vi "Read-Write Program File.vi"(0 "configuration file path":path=path "C:/ProgramData/PVI Systems/Vision Inspection System/Config.ini", 1 "Program in":T2={"Raw Logging Configuration"={"Log File Base Path"=path "", "Enable Log File"=FALSE}, "Sequence"={"Start RPM"=10.0, "End RPM"=9600.0, "# RPM Steps"=1, "Dwell (s)"=2.0, "Start L-value / Resist"=0, "End L-value/Resist"=0, "# L-value/Resist Steps"=0, "Steady State +/-RPM"=10.0, "Enable Steady State +/- RPM"=FALSE, "Steady State Window (s)"=10.0, "Enable Steady State Max Wait"=FALSE, "Max Settle Time (s)"=10.0, "Enable Temperature Rest"=FALSE, "Rest TC2 threshold (degF)"=2.0, "Enable Max Time Rest"=FALSE, "Max Rest Time (s)"=10.0, "Rest RPM"=2.0, "RPM Ramp (rpm/s)"=10.0, "Resistance Motor Mode"=enum."v1 Bike"}, "Summary  CSV Log Configuration"={"Report  CSV File Path"=path "C:/Users/nlim/Documents/LabVIEW Data/Logged Data.tdms", "Enable Report CSV File"=FALSE}, "CSV Log Info"={"Report Title"="", "Time Stamp"=timestamp(0 s since 1904-01-01), "Serial Number"="", "Initial Temperature"=0.0, "Comments"=""}, "Table"=[]} {"Sequence"."RPM Ramp (rpm/s)" min=0.0 format="%#_6f"; "Sequence"."Rest RPM" min=0.0 format="%.1f"; "Sequence"."Max Rest Time (s)" min=0.0 format="%.1f"; "Sequence"."Rest TC2 threshold (degF)" format="%.1f"; "Sequence"."Max Settle Time (s)" min=0.0 format="%.1f"; "Sequence"."Steady State Window (s)" min=0.0 format="%.1f"; "Sequence"."Steady State +/-RPM" min=0.0 format="%.1f"; "Sequence"."# L-value/Resist Steps" min=1; "Sequence"."End L-value/Resist" min=0 max=100; "Sequence"."Start L-value / Resist" min=0 max=100; "Sequence"."Dwell (s)" min=0.0 format="%#_6f"; "Sequence"."# RPM Steps" min=1; "Sequence"."End RPM" min=0.0 max=200.0 format="%#_6f"; "Sequence"."Start RPM" min=0.0 max=200.0 format="%#_6f"}, 2 "Mode":T1=enum."Write", 3 "error in":errorcluster) -> (7 "Config File Path":path=path "C:/ProgramData/PVI Systems/Vision Inspection System/Config.ini", 8 "Program out":T2={"Raw Logging Configuration"={"Log File Base Path"=path "", "Enable Log File"=FALSE}, "Sequence"={"Start RPM"=10.0, "End RPM"=9600.0, "# RPM Steps"=1, "Dwell (s)"=2.0, "Start L-value / Resist"=0, "End L-value/Resist"=0, "# L-value/Resist Steps"=0, "Steady State +/-RPM"=10.0, "Enable Steady State +/- RPM"=FALSE, "Steady State Window (s)"=10.0, "Enable Steady State Max Wait"=FALSE, "Max Settle Time (s)"=10.0, "Enable Temperature Rest"=FALSE, "Rest TC2 threshold (degF)"=2.0, "Enable Max Time Rest"=FALSE, "Max Rest Time (s)"=10.0, "Rest RPM"=2.0, "RPM Ramp (rpm/s)"=10.0, "Resistance Motor Mode"=enum."v1 Bike"}, "Summary  CSV Log Configuration"={"Report  CSV File Path"=path "C:/Users/nlim/Documents/LabVIEW Data/Logged Data.tdms", "Enable Report CSV File"=FALSE}, "CSV Log Info"={"Report Title"="", "Time Stamp"=timestamp(0 s since 1904-01-01), "Serial Number"="", "Initial Temperature"=0.0, "Comments"=""}, "Table"=[]} {"Sequence"."RPM Ramp (rpm/s)" min=0.0 format="%#_6f"; "Sequence"."Rest RPM" min=0.0 format="%.1f"; "Sequence"."Max Rest Time (s)" min=0.0 format="%.1f"; "Sequence"."Rest TC2 threshold (degF)" format="%.1f"; "Sequence"."Max Settle Time (s)" min=0.0 format="%.1f"; "Sequence"."Steady State Window (s)" min=0.0 format="%.1f"; "Sequence"."Steady State +/-RPM" min=0.0 format="%.1f"; "Sequence"."# L-value/Resist Steps" min=1; "Sequence"."End L-value/Resist" min=0 max=100; "Sequence"."Start L-value / Resist" min=0 max=100; "Sequence"."Dwell (s)" min=0.0 format="%#_6f"; "Sequence"."# RPM Steps" min=1; "Sequence"."End RPM" min=0.0 max=200.0 format="%#_6f"; "Sequence"."Start RPM" min=0.0 max=200.0 format="%#_6f"}, 10 "error out":errorcluster)   [LabVIEW 2015, in "Config Module.lvlib"]
uses:
  Config Module.lvlib
  Settings/Program Cluster.ctl
  Logging/Logging Configuration.ctl
  Settings/Sequence Cluster.ctl
  Resistance Motor/Resistance Mode Enum.ctl
  controls/CSV Log Cluster.ctl
  controls/CSV Log Info Cluster.ctl
  Controls/Config File Operation Enum.ctl
  XML Config/XML Config.lvlib
  Logging/Logging.lvlib
  Settings/Settings.lvlib
panel:
  # "Settled when"
  # "RPM is within"
  # "RPM of set RPM for last"
  # "seconds"
  # "OR"
  # "seconds since last step change"
  # "More than"
  # "Rest at end of each step at"
  # "RPM until"
  # "TC2 temperature is below"
  # "deg F"
  # "OR"
  # "seconds have elapsed"
  # "More than"
  # "Settled when"
  # "RPM is within"
  # "RPM of set RPM for last"
  # "seconds"
  # "OR"
  # "seconds since last step change"
  # "More than"
  # "Rest at end of each step at"
  # "RPM until"
  # "TC2 temperature is below"
  # "deg F"
  # "OR"
  # "seconds have elapsed"
  # "More than"
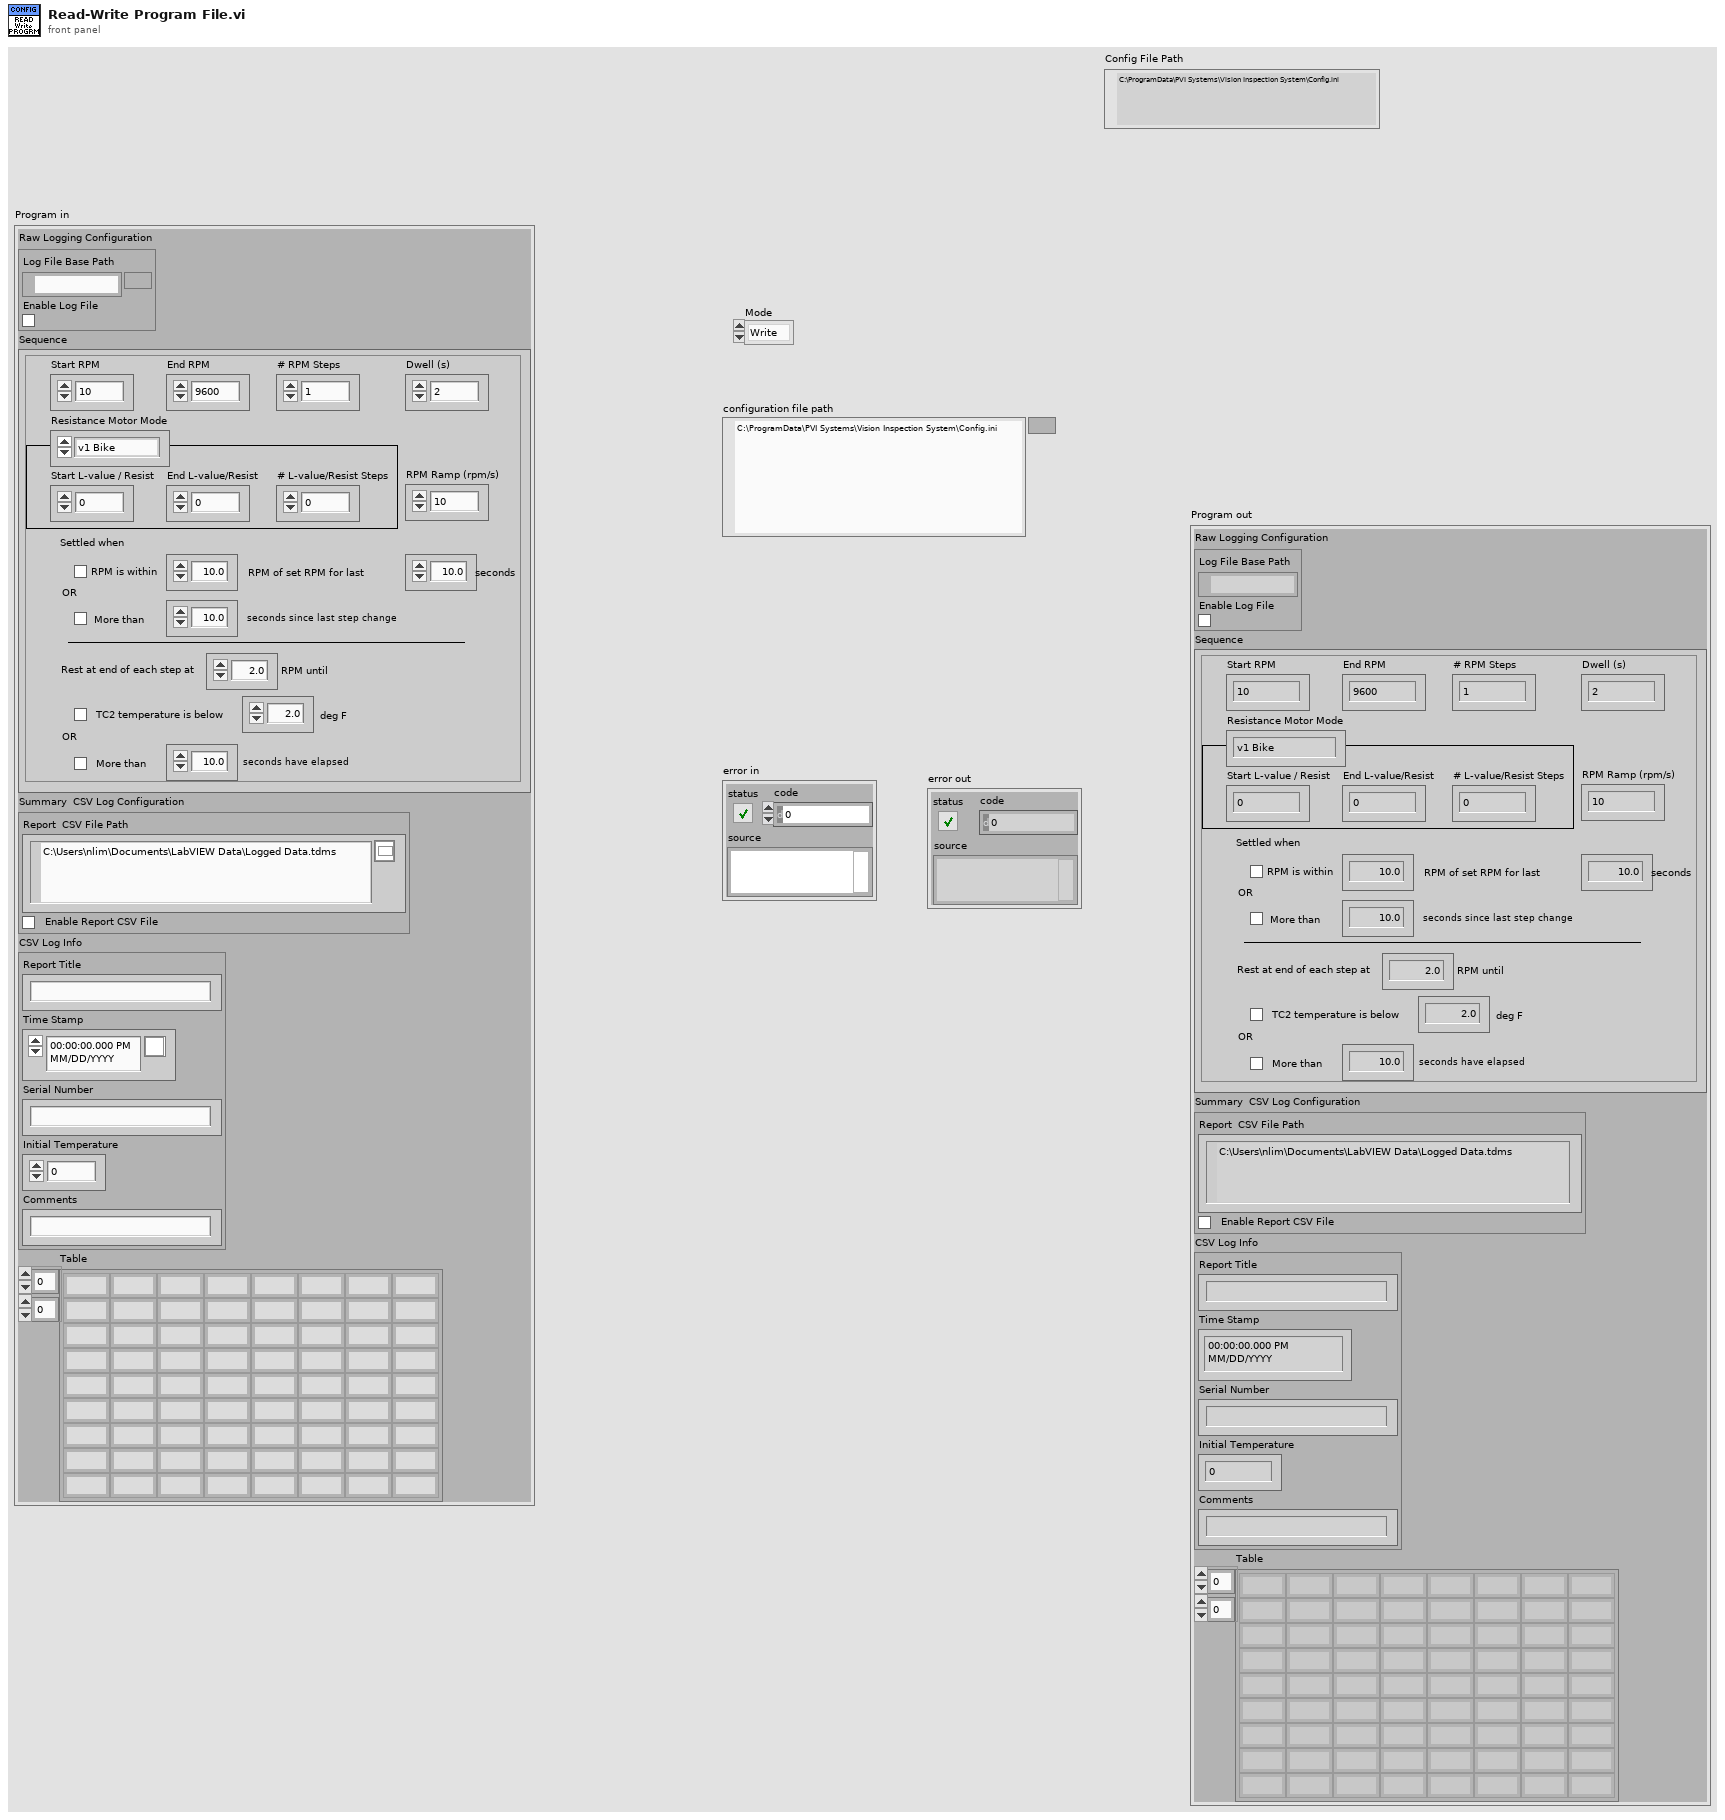
[diagram p1: front panel]
types:
  T1 = typedef "Config Module.lvlib/Config File Operation Enum.ctl" = enum16{"Read", "Write"}
  T2 = typedef "Settings.lvlib/Program Cluster.ctl" = cluster{"Raw Logging Configuration":T3, "Sequence":T4, "Summary  CSV Log Configuration":T6, "CSV Log Info":T7, "Table":string[][]}
  T3 = typedef "Logging.lvlib/Logging Configuration.ctl" = cluster{"Log File Base Path":path, "Enable Log File":bool}
  T4 = typedef "Sequence Cluster.ctl" = cluster{"Start RPM":dbl, "End RPM":dbl, "# RPM Steps":i32, "Dwell (s)":dbl, "Start L-value / Resist":i32, "End L-value/Resist":i32, "# L-value/Resist Steps":i32, "Steady State +/-RPM":dbl, "Enable Steady State +/- RPM":bool, "Steady State Window (s)":dbl, "Enable Steady State Max Wait":bool, "Max Settle Time (s)":dbl, "Enable Temperature Rest":bool, "Rest TC2 threshold (degF)":dbl, "Enable Max Time Rest":bool, "Max Rest Time (s)":dbl, "Rest RPM":dbl, "RPM Ramp (rpm/s)":dbl, "Resistance Motor Mode":T5}
  T5 = typedef "Resistance Mode Enum.ctl" = enum16{"v1 Bike", "v1.5 Bike", "Disabled"}
  T6 = typedef "CSV Log Cluster.ctl" = cluster{"Report  CSV File Path":path, "Enable Report CSV File":bool}
  T7 = typedef "CSV Log Info Cluster.ctl" = cluster{"Report Title":string, "Time Stamp":timestamp, "Serial Number":string, "Initial Temperature":dbl, "Comments":string}
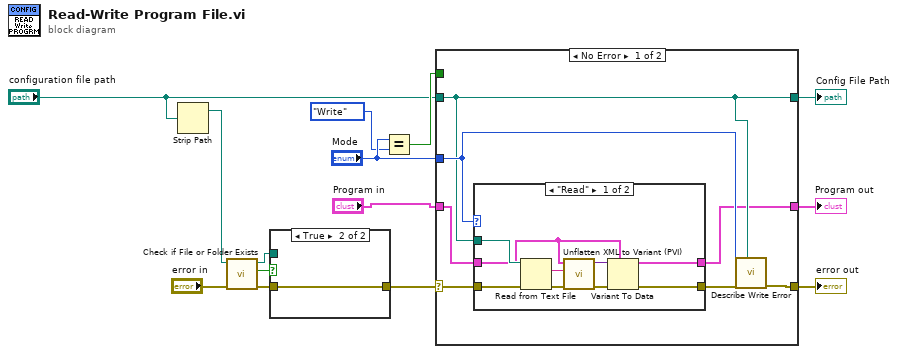
[diagram p0: block diagram]
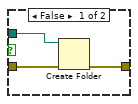
[diagram p2: hidden frame]
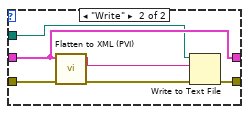
[diagram p3: hidden frame]
diagram:
  n1 = Strip Path(path="configuration file path") -> (stripped path=w9:path)  [unwired: 1 out]
  n2 = call <vilib>:"Check if File or Folder Exists.vi"("error in (no error)"="error in", "path"=w9) -> ("error out"=w6:errorcluster, "file or folder exists?"=w7:bool, "dup path"=w4:path)  [unwired: 7 in]
  n3 = case shown="True" w7 {
    tunnel: w6 -> [w17 w18]
    tunnel: [w16 w18] -> w5
    tunnel: w4 -> [w15 _]
    frame False {
      n4 = Create Folder(path (use dialog)=w15, error in=w17) -> (error out=w16:errorcluster)  [unwired: 1 in, 2 out]
    }
    frame True {
    }
  }
  n5 = Equal?(x="Mode", y=Config_File_Operation_Enum."Write" ("Mode")) -> (x = y?=w10:bool)
  n6 = case shown="No Error" w5 {
    selector: w5 -> [w21 w42]
    tunnel: [w25 w42] -> w14
    tunnel: "configuration file path" -> [w22 w43]
    tunnel: "Program in" -> [w23 w41]
    tunnel: [w22 w43] -> w13
    tunnel: "Mode" -> [w24 _]
    tunnel: w10 -> [_ _]
    tunnel: [w19 w41] -> w1
    frame No Error {
      n7 = case shown="\"Read\"" w24 {
        tunnel: [w28 w39] -> w19
        tunnel: w23 -> [w30 w39]
        tunnel: w21 -> [w33 w40]
        tunnel: w22 -> [w34 w37]
        tunnel: [w26 w36] -> w20
        frame "Read" {
          n8 = Read from Text File(file (use dialog)=w34, error in=w33) -> (text=w31:string, error out=w32:errorcluster)  [unwired: 2 in, 2 out]
          n9 = call "Unflatten XML to Variant (PVI).vi"("error in (no error)"=w32, "XML"=w31, "Variant in (for type and default data)"=w30) -> ("error out"=w27:errorcluster, "Variant out"=w29:variant)  [unwired: 7 in]
          n10 = Variant To Data(error in=w27, type=w30, Variant=w29) -> (data=w28:T2, error out=w26:errorcluster)
        }
        frame "Write" {
          n11 = call "Flatten to XML (PVI).vi"("error in (no error)"=w40, "Variant"=w39) -> ("error out"=w38:errorcluster, "XML"=w35:string)  [unwired: 8 in]
          n12 = Write to Text File(file (use dialog)=w37, text=w35, error in=w38) -> (error out=w36:errorcluster)  [unwired: 1 in, 2 out]
        }
      }
      n13 = call "Describe Write Error.vi"("Config File Path"=w22, "error in (no error)"=w20, "Mode"=w24) -> ("error out"=w25:errorcluster)  [unwired: 8 in]
    }
    frame Error {
    }
  }
  "error out" <- w14
  "Config File Path" <- w13
  "Program out" <- w1
